vi "getSeperator.vi"(10 "Channel Seperator (\"\")":string="Channel", 11 "Command":string) -> (2 "Channel":string, 3 "Seperator (e.g. \"Channel1\")":string="Channel1")   [LabVIEW 2011]
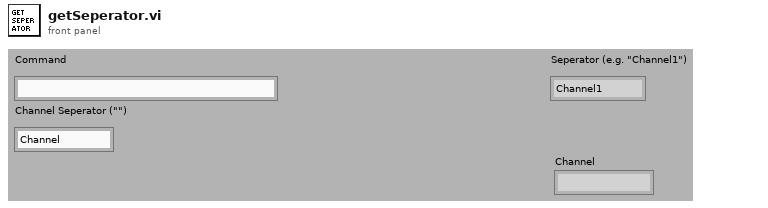
[diagram p1: front panel]
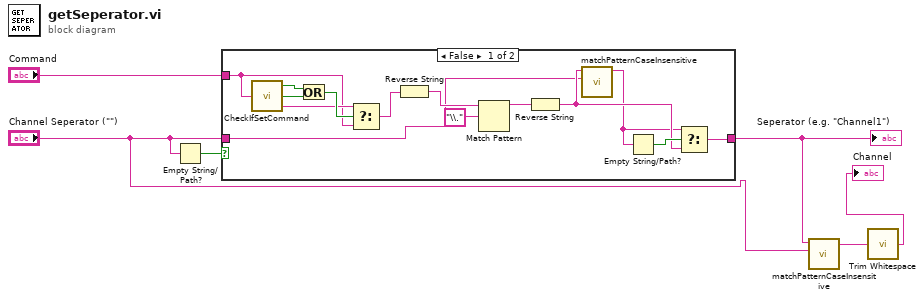
[diagram p0: block diagram]
diagram:
  n1 = Empty String/Path?(string/path="Channel Seperator (\"\")") -> (empty?=w5:bool)
  n2 = case shown="False" w5 {
    tunnel: "Command" -> [w16 _]
    tunnel: "Channel Seperator (\"\")" -> [w8 w21]
    tunnel: [w10 w21] -> w4
    frame False {
      n3 = call "CheckIfSetCommand.vi"("Command"=w16) -> ("setCommand?"=w20:bool, "getCommand?"=w19:bool, "variable"=w17:string)
      n4 = Or(x=w20, y=w19) -> (x .or. y?=w18:bool)
      n5 = Select(t=w17, s=w18, f=w16) -> (s? t:f=w12:string)
      n6 = Reverse String(1:w12) -> (0:w15:string)
      n7 = Match Pattern(string=w15, regular expression="\\.") -> (before substring=w13:string)  [unwired: 1 in, 3 out]
      n8 = Reverse String(1:w13) -> (0:w9:string)
      n9 = call "matchPatternCaseInsensitive.vi"("String"=w8, "Command 4"=w9) -> ("after"=w7:string)  [unwired: 7 in, 2 out]
      n10 = Empty String/Path?(string/path=w7) -> (empty?=w11:bool)
      n11 = Select(t=w7, s=w11, f=w9) -> (s? t:f=w10:string)
    }
    frame True {
    }
  }
  "Seperator (e.g. \"Channel1\")" <- w4
  n12 = call "matchPatternCaseInsensitive.vi"("String"="Channel Seperator (\"\")", "Command 4"=w4) -> ("after"=w2:string)  [unwired: 7 in, 2 out]
  n13 = call "Trim Whitespace.vi"("string"=w2) -> ("trimmed string"=→"Channel":string)  [unwired: 1 in]
